vi "Using TC01.vi"() -> ()   [LabVIEW 2017]
panel:
  in  "Stop Button":bool
  out "Numeric Indicator":dbl format="%.1g"
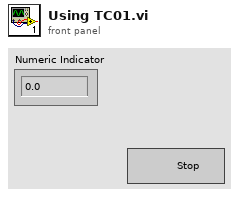
[diagram p1: front panel]
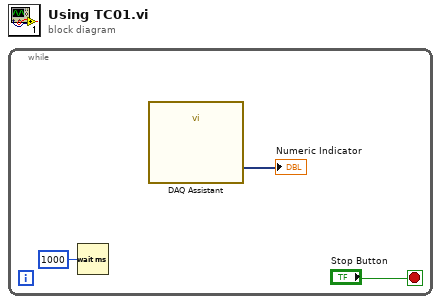
[diagram p0: block diagram]
diagram:
  n1 = while {
    stop <- "Stop Button" stop-if-true
    n2 = Wait (ms)(milliseconds to wait=u32 1000) -> ()  [unwired: 1 out]
    n3 = call "DAQ Assistant"() -> ("data"=→"Numeric Indicator":dynamicdata)  [unwired: 17 in, 2 out]
  }
